vi "Check Guest History.vi"(0 "Guest Manager Model in":refnum<class "Guest Manager Model.lvclass">, 5 "Guest Contact Number In":string caption="Guest Contact Number", 11 "error in (no error)":errorcluster) -> (4 "Guest Manager Model out":refnum<class "Guest Manager Model.lvclass">, 15 "error out":errorcluster)   [LabVIEW 2023, in "Guest Manager Model.lvlib" / "Guest Manager Model.lvclass"]
uses:
  Guest Manager Model.lvclass
  Guest Manager Model.lvclass/Guest Manager Model.ctl
  Interfaces/Incoming Rooms Manager Model Interface Messages/Check Guest History Msg/Check Guest History Msg.lvclass
  <vilib>/ActorFramework/Actor/Actor.lvclass
  C:/Users/bhaghyaraj/Trainings/NI Actor Framework/SDLC/Model Base/Model Base/Model Base.lvclass
  C:/Program Files/National Instruments/LabVIEW 2023/vi.lib/ActorFramework/Actor/Actor.lvclass
  C:/Users/bhaghyaraj/Trainings/NI Actor Framework/SDLC/Interfaces/Model Base/Incoming Model Base Interface.lvclass
  C:/Users/bhaghyaraj/Trainings/NI Actor Framework/SDLC/Guest Manager Model/Guest Manager Model/Guest Manager Model.lvclass
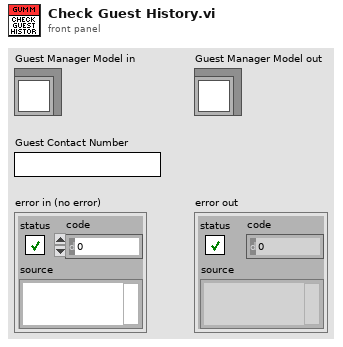
[diagram p1: front panel]
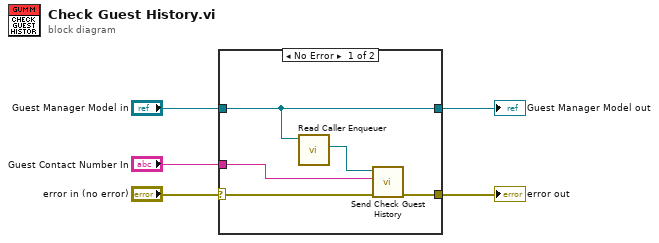
[diagram p0: block diagram]
diagram:
  n1 = case shown="No Error" "error in (no error)" {
    selector: "error in (no error)" -> [w10 w12]
    tunnel: [w9 w12] -> w4
    tunnel: [w8 w11] -> w2
    tunnel: "Guest Manager Model in" -> [w8 w11]
    tunnel: "Guest Contact Number In" -> [w6 _]
    frame No Error {
      n2 = call <vilib>:"Read Caller Enqueuer.vi"("Actor"=w8) -> ("Caller Enqueuer"=w7:refnum<class "Message Enqueuer.lvclass">)  [unwired: 10 in]
      n3 = call "Send Check Guest History.vi"("error in (no error)"=w10, "Guest Contact Number In"=w6, "Message Enqueuer"=w7) -> ("error out"=w9:errorcluster)  [unwired: 7 in, 1 out]
    }
    frame Error {
    }
  }
  "error out" <- w4
  "Guest Manager Model out" <- w2
